vi "Initialize.vi"(8 "error in (no error)":errorcluster, 11 "Component Settings Editor in":refnum<class "Component Settings Editor.lvclass">) -> (0 "error out":errorcluster, 3 "Component Settings Editor out":refnum<class "Component Settings Editor.lvclass">)   [LabVIEW 2017, in "DSF Core.lvlib" / "Component Settings Editor.lvclass"]
uses:
  Component Settings Editor.lvclass
  C:/Git/DSF/Core/Classes/User Interface/User Interface.lvclass
  User Interface.lvclass
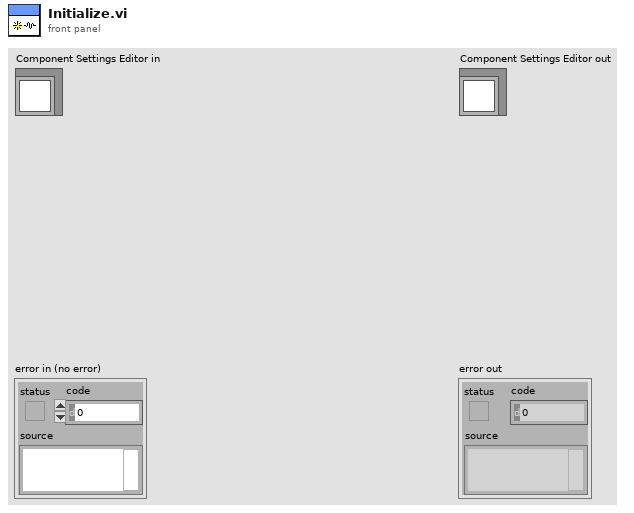
[diagram p1: front panel]
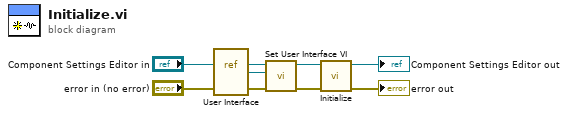
[diagram p0: block diagram]
diagram:
  n1 = vi-ref "User Interface.vi"() -> (w7:refnum<vi>)
  n2 = call "Set User Interface VI.vi"("error in (no error)"="error in (no error)", "vi"=w7, "User Interface in"="Component Settings Editor in") -> ("error out"=w4:errorcluster, "User Interface out"=w3:refnum<class "Component Settings Editor.lvclass">)  [unwired: 7 in]
  n3 = call-parent "Initialize.vi"("error in (no error)"=w4, "User Interface in"=w3) -> ("error out"=→"error out":errorcluster, "User Interface out"=→"Component Settings Editor out":refnum<class "Component Settings Editor.lvclass">)  [unwired: 8 in]
